vi "hpanel_DO_change_hydraharp_settings.vi"(8 "error in (no error)":errorcluster, 9 "Mode":T5 items=["T2"=2, "T3"=3], 10 "Hydraharp Settings":T1 {"CH 8"."ch_offs" min=-99999 max=99999 step=1; "CH 8"."ch_ZeroX" min=0 max=20 step=1; "CH 8"."ch_level" min=0 max=800 step=1; "CH 7"."ch_offs" min=-99999 max=99999 step=1; "CH 7"."ch_ZeroX" min=0 max=20 step=1; "CH 7"."ch_level" min=0 max=800 step=1; "CH 6"."ch_offs" min=-99999 max=99999 step=1; "CH 6"."ch_ZeroX" min=0 max=20 step=1; "CH 6"."ch_level" min=0 max=800 step=1; "CH 5"."ch_offs" min=-99999 max=99999 step=1; "CH 5"."ch_ZeroX" min=0 max=20 step=1; "CH 5"."ch_level" min=0 max=800 step=1; "binning" min=0 max=10 step=1; "CH 4"."ch_offs" min=-99999 max=99999 step=1; "CH 4"."ch_ZeroX" min=0 max=20 step=1; "CH 4"."ch_level" min=0 max=800 step=1; "CH 3"."ch_offs" min=-99999 max=99999 step=1; "CH 3"."ch_ZeroX" min=0 max=20 step=1; "CH 3"."ch_level" min=0 max=800 step=1; "CH 2"."ch_offs" min=-99999 max=99999 step=1; "CH 2"."ch_ZeroX" min=0 max=20 step=1; "CH 2"."ch_level" min=0 max=800 step=1; "CH 1"."ch_offs" min=-99999 max=99999 step=1; "CH 1"."ch_ZeroX" min=0 max=20 step=1; "CH 1"."ch_level" min=0 max=800 step=1; "Sync Settings"."snc_offs" min=-99999 max=99999 step=1; "Sync Settings"."snc_ZeroX" min=0 max=20 step=1; "Sync Settings"."snc_level" min=0 max=800 step=10}, 11 "hydraharp_panel in":refnum<class "hydraharp_panel.lvclass">) -> (0 "error out":errorcluster, 3 "hydraharp_panel out":refnum<class "hydraharp_panel.lvclass">)   [LabVIEW 2015, in "hydraharp_panel.lvclass"]
uses:
  hydraharp_panel.lvclass
  hpanel_acq_modes.ctl
  hpanel_hydraharp_settings.ctl
  hpanel_sync_settings.ctl
  hpanel_sync_div.ctl
  hpanel_channel_settings.ctl
  hydraharp/hydraharp.lvclass
  hydraharp/hydraharp.lvclass/hydraharp.ctl
  UI/panel_class/panel.lvclass
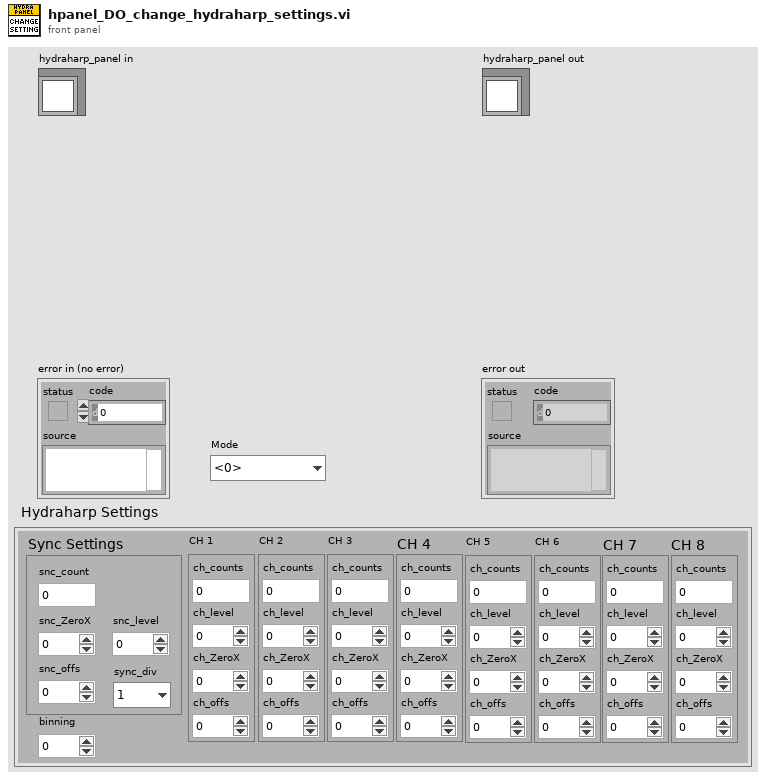
[diagram p1: front panel]
types:
  T1 = typedef "hpanel_hydraharp_settings.ctl" = cluster{"Sync Settings":T2, "CH 1":T4, "CH 2":T4, "CH 3":T4, "CH 4":T4, "binning":i32, "CH 5":T4, "CH 6":T4, "CH 7":T4, "CH 8":T4}
  T2 = typedef "hpanel_sync_settings.ctl" = cluster{"snc_count":i32, "snc_level":i32, "snc_ZeroX":i32, "snc_offs":i32, "sync_div":T3}
  T3 = typedef "hpanel_sync_div.ctl" = enum16{"1", "2", "4", "8"}
  T4 = typedef "hpanel_channel_settings.ctl" = cluster{"ch_counts":i32, "ch_level":i32, "ch_ZeroX":i32, "ch_offs":i32}
  T5 = typedef "hpanel_acq_modes.ctl" = u16
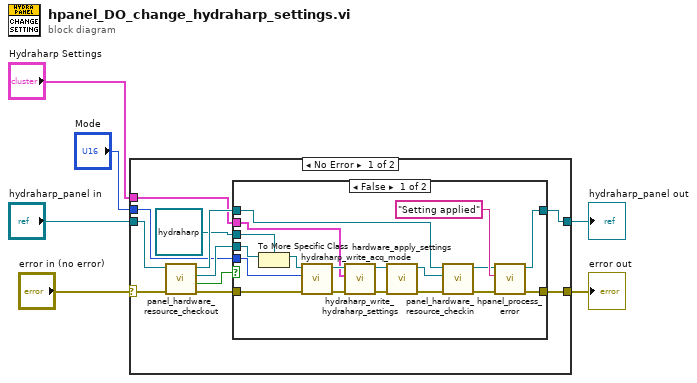
[diagram p0: block diagram]
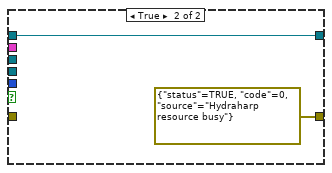
[diagram p2: hidden frame]
diagram:
  n1 = case shown="No Error" "error in (no error)" {
    selector: "error in (no error)" -> [w16 w39]
    tunnel: [w13 w39] -> w5
    tunnel: [w7 w38] -> w3
    tunnel: "hydraharp_panel in" -> [w17 w38]
    tunnel: "Mode" -> [w9 _]
    tunnel: "Hydraharp Settings" -> [w8 _]
    frame No Error {
      n2 = call "panel_hardware_resource_checkout.vi"("error in (no error)"=w16, "panel in"=w17) -> ("error out"=w14:errorcluster, "timed out?"=w15:bool, "hardware.lvclass"=w11:refnum<class "hardware.lvclass">, "panel out"=w12:refnum<class "hydraharp_panel.lvclass">)  [unwired: 6 in]
      n3 = case shown="False" w15 {
        tunnel: w14 -> [w33 _]
        tunnel: [w18 errorcluster {"status"=TRUE, "code"=0, "source"="Hydraharp resource busy"} ("error out")] -> w13
        tunnel: w12 -> [w27 w36]
        tunnel: w11 -> [w34 _]
        tunnel: refnum<class "hydraharp.lvclass"> refnum ("hydraharp.lvclass") -> [w35 _]
        tunnel: w9 -> [w29 _]
        tunnel: w8 -> [w28 _]
        tunnel: [w19 w36] -> w7
        frame False {
          n4 = To More Specific Class(target class=w35, reference=w34) -> (specific class reference=w32:refnum<class "hydraharp.lvclass">)  [unwired: 1 in, 1 out]
          n5 = call "hydraharp_write_acq_mode.vi"("error in (no error)"=w33, "Mode"=w29, "hydraharp in"=w32) -> ("error out"=w30:errorcluster, "hydraharp out"=w31:refnum<class "hydraharp.lvclass">)  [unwired: 7 in]
          n6 = call "hydraharp_write_hydraharp_settings.vi"("error in (no error)"=w30, "Hydraharp Settings"=w28, "hydraharp in"=w31) -> ("error out"=w24:errorcluster, "hydraharp out"=w23:refnum<class "hydraharp.lvclass">)  [unwired: 7 in]
          n7 = call-dynamic "hardware_apply_settings.vi"("error in (no error)"=w24, "hydraharp in"=w23) -> ("error out"=w25:errorcluster, "hydraharp out"=w26:refnum<class "hydraharp.lvclass">)  [unwired: 8 in]
          n8 = call "panel_hardware_resource_checkin.vi"("error in (no error)"=w25, "hardware.lvclass"=w26, "panel in"=w27) -> ("error out"=w22:errorcluster, "panel out"=w20:refnum<class "hydraharp_panel.lvclass">)  [unwired: 7 in]
          n9 = call "hpanel_process_error.vi"("error in (no error)"=w22, "No Error Message"="Setting applied" ("String"), "hydraharp_panel in"=w20) -> ("error out"=w18:errorcluster, "hydraharp_panel out"=w19:refnum<class "hydraharp_panel.lvclass">)  [unwired: 7 in]
        }
        frame True {
        }
      }
    }
    frame Error {
    }
  }
  "error out" <- w5
  "hydraharp_panel out" <- w3
